vi "dvp Vi Get Color Solution Sel.vi"(10 "pColorSolutionSel":u32, 11 "handle":u32) -> (2 "pColorSolutionSel out":u32, 3 "function return":u32(ring))   [LabVIEW 2018, in "LabViewDVPCamera.lvlib"]
doc: "LabviewDvp2Api dvpStatus dvpViGetColorSolutionSel(dvpHandle handle, dvpUint32 *pColorSolutionSel);"
uses:
  LabViewDVPCamera.lvlib
  LabViewDVPCamera/LabViewDVPCamera.dll
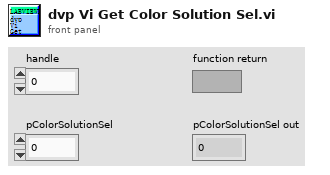
[diagram p1: front panel]
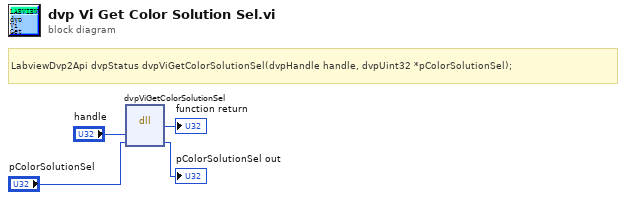
[diagram p0: block diagram]
diagram:
  # "LabviewDvp2Api dvpStatus dvpViGetColorSolutionSel(dvpHandle handle, dvpUint32 *pColorSolutionSel);"
  n1 = dll-call lib="C:/Program Files (x86)/DVP2 Labview cn 64/Sample/LabViewDVPCamera/LabViewDVPCamera.*" fn="dvpViGetColorSolutionSel"("handle"="handle", "pColorSolutionSel"="pColorSolutionSel") -> (→"function return":u32, "pColorSolutionSel"=→"pColorSolutionSel out":u32)  [unwired: 4 in, 2 out]
